vi "stage_idling.vi"(9 "num":u8, 10 "pos":dbl, 11 "Array":dbl[](array[numeric])) -> ()   [LabVIEW 2019, in "dummyStage.lvlib" / "dummyStage.lvclass"]
uses:
  dummyStage.lvclass
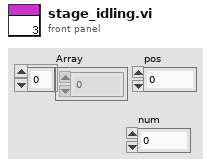
[diagram p1: front panel]
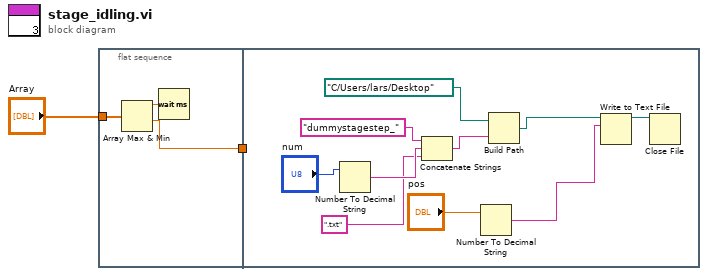
[diagram p0: block diagram]
diagram:
  n1 = flat-sequence {
    tunnel: "Array" -> [w4]
    tunnel: [w3] -> w1
    tunnel: w1 -> [_]
    frame #0 {
      n2 = Array Max & Min(array=w4) -> (max value=w5:dbl, min value=w3:dbl)  [unwired: 2 out]
      n3 = Wait (ms)(milliseconds to wait=w5) -> ()  [unwired: 1 out]
    }
    frame #1 {
      n4 = Number To Decimal String(number="num") -> (decimal integer string=w9:string)  [unwired: 1 in]
      n5 = Concatenate Strings("dummystagestep_", w9, ".txt") -> (w7:string)
      n6 = Number To Decimal String(number="pos") -> (decimal integer string=w13:string)  [unwired: 1 in]
      n7 = Build Path(base path=path "C:/Users/lars/Desktop" ("file (use dialog)"), name or relative path=w7) -> (appended path=w6:path)
      n8 = Write to Text File(file (use dialog)=w6, text=w13) -> (refnum out=w14:refnum<file>)  [unwired: 2 in, 2 out]
      n9 = Close File(refnum=w14) -> ()  [unwired: 1 in, 2 out]
    }
  }
